vi "UpdateUserTable.vi"(8 "Error in":errorcluster caption="Error in (no error)", 11 "User Table":refnum<vi>) -> (0 "error out":errorcluster)   [LabVIEW 2017, in "Login-UI.lvlib"]
uses:
  Login-UI.lvlib
  <userlib>/NEVSTOP-Programming-Palette/Configuration/ClusterCfgTable/ClusterCfgTable_nevstop.lvlib
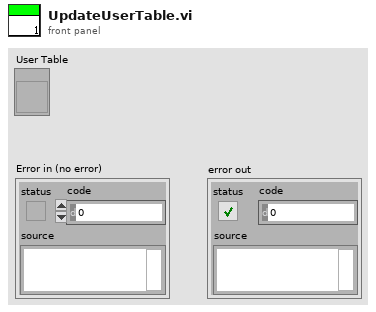
[diagram p1: front panel]
types:
  T1 = typedef "Login-UI.lvlib/User-Info.ctl" = cluster{"UserName":string, "Password":string, "Role":T2}
  T2 = typedef "Login-UI.lvlib/User-Role.ctl" = enum16{"INVALID", "Operator", "Engineer", "Admin"}
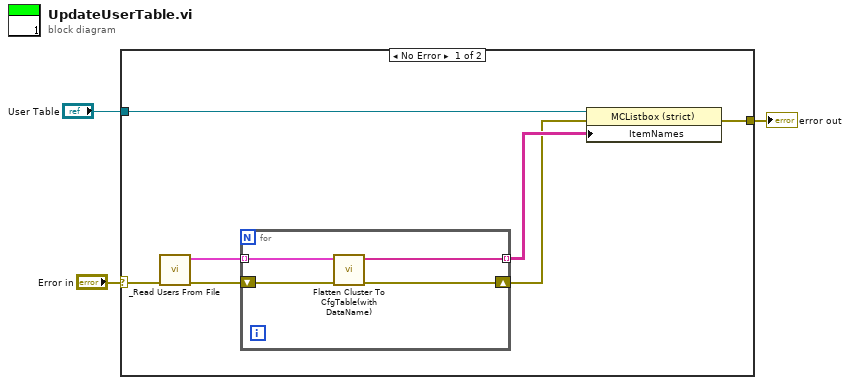
[diagram p0: block diagram]
diagram:
  n1 = case shown="No Error" "Error in" {
    selector: "Error in" -> [w5 w15]
    tunnel: "User Table" -> [w10 _]
    tunnel: [w4 w15] -> w1
    frame No Error {
      n2 = call "_Read Users From File.vi"("Error in"=w5) -> ("Error out"=w7:errorcluster, "Array"=w9:T1[])  [unwired: 9 in]
      n3 = for {
        tunnel: w9 -> [w14] mode=indexing
        tunnel: [w13] -> w8 mode=indexing
        shift-right: [w11] -> w6
        shift-left: w7 -> [w12]
        n4 = call <userlib>:"Flatten Cluster To CfgTable(with DataName).vi"("error in (no error)"=w12, "Cluster Configuration Typedef"=w14) -> ("error out"=w11:errorcluster, "CfgTable Row"=w13:string[])  [unwired: 7 in, 1 out]
      }
      n5 = property class="MCListbox (strict)"(reference=w10, error in=w6, "ItemNames"=w8) -> (error out=w4:errorcluster)  [unwired: 1 out]
    }
    frame Error {
    }
  }
  "error out" <- w1
